vi "Convert Hex String to Array.vi"(7 "Hex String In":string) -> (8 "Hex Array Out":u8[](array[numeric]) format="%.0x")   [LabVIEW 2019, in "GEA2_Toolkit.lvlib"]
uses:
  library/GEA2_Toolkit.lvlib
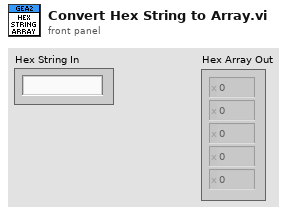
[diagram p1: front panel]
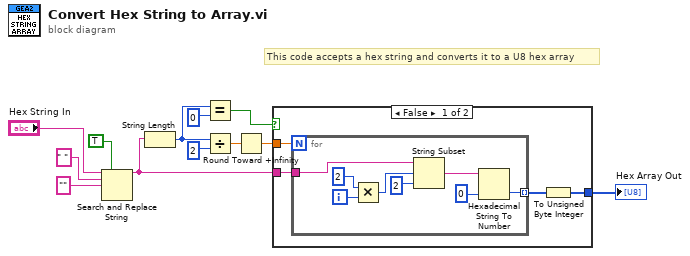
[diagram p0: block diagram]
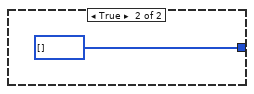
[diagram p2: hidden frame]
diagram:
  # "This code accepts a hex string and converts it to a U8 hex array"
  n1 = Search and Replace String(replace all?=TRUE ("replace all? (F)"), input string="Hex String In", search string=" ", replace string="" ("replace string (\"\")")) -> (result string=w10:string)  [unwired: 4 in, 3 out]
  n2 = String Length(string=w10) -> (length=w6:i32)
  n3 = Equal?(x=w6, y=0) -> (x = y?=w8:bool)
  n4 = Divide(x=w6, y=2) -> (x/y=w3:dbl)
  n5 = Round Toward +Infinity(x=w3) -> (ceil(x): smallest int >= x=w4:dbl)
  n6 = case shown="False" w8 {
    tunnel: w10 -> [w16 _]
    tunnel: [w15 u8[] []] -> w1
    tunnel: w4 -> [w13 _]
    frame False {
      n7 = for {
        N: w13 -> [_]
        tunnel: w16 -> [w22]
        tunnel: [w17] -> w14 mode=indexing
        i -> [w24]
        n8 = Multiply(x=2, y=w24) -> (x*y=w21:i32)
        n9 = String Subset(string=w22, offset (0)=w21, length (rest)=2 ("length (rest)")) -> (substring=w18:string)
        n10 = Hexadecimal String To Number(string=w18, default (0uL)=u32 0 ("default (0 U32)")) -> (number=w17:u32)  [unwired: 1 in, 1 out]
      }
      n11 = To Unsigned Byte Integer(number=w14) -> (unsigned 8bit integer=w15:u8[])
    }
    frame True {
    }
  }
  "Hex Array Out" <- w1
